vi "Write use TDMS_.vi"(8 "error in":errorcluster, 10 "use TDMS?":bool=TRUE, 11 "TDMS in":refnum<class "TDMS.lvclass">) -> (0 "error out":errorcluster, 3 "TDMS out":refnum<class "TDMS.lvclass">)   [LabVIEW 2017, in "Report_lib.lvlib" / "TDMS.lvclass"]
uses:
  TDMS.lvclass
  TDMS.lvclass/TDMS.ctl
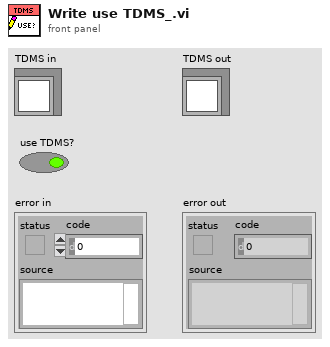
[diagram p1: front panel]
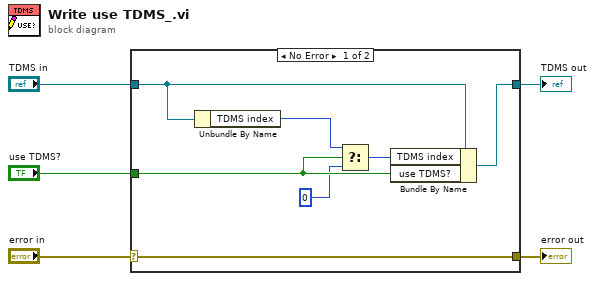
[diagram p0: block diagram]
diagram:
  n1 = case shown="No Error" "error in" {
    selector: "error in" -> [w12 w13]
    tunnel: [w12 w13] -> w4
    tunnel: [w11 w14] -> w2
    tunnel: "TDMS in" -> [w10 w14]
    tunnel: "use TDMS?" -> [w9 _]
    frame No Error {
      n2 = Unbundle By Name(w10) -> ("TDMS index"=w8:i32)
      n3 = Select(t=w8, s=w9, f=0) -> (s? t:f=w7:i32)
      n4 = Bundle By Name(cluster=w10, "TDMS index"=w7, "use TDMS?"=w9) -> (w11:refnum<class "TDMS.lvclass">)
    }
    frame Error {
    }
  }
  "error out" <- w4
  "TDMS out" <- w2
